vi "Cleanup.vi"(8 "error in (no error)":errorcluster, 11 "LV-Term App in":refnum<class "LV-Term App.lvclass">) -> (0 "error out":errorcluster)   [LabVIEW 2020, in "LV-Term.lvlib" / "LV-Term App.lvclass"]
uses:
  LV-Term App.lvclass
  LV-Term App.lvclass/LV-Term App.ctl
  <vilib>/IlluminatedG/IG OOPanel/OOPanel/Manager/Manager.lvclass
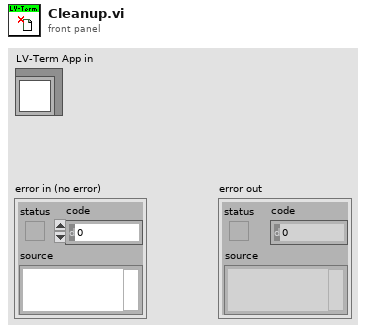
[diagram p1: front panel]
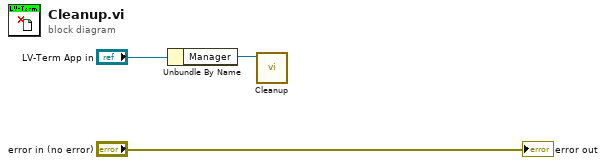
[diagram p0: block diagram]
diagram:
  n1 = Unbundle By Name("LV-Term App in") -> ("Manager"=w1:refnum<class "Manager.lvclass">)
  n2 = call <vilib>:"Cleanup.vi"("Manager in"=w1) -> ()  [unwired: 8 in, 3 out]
  "error out" <- "error in (no error)"
